vi "Get Count LED Settings From Recipe.vi"(11 "Test Recipe in":refnum<class "Test Recipe.lvclass">) -> (1 "Threshold Values":T1={"Red Range"={"Lower value"=0, "Upper value"=95}, "Green Range"={"Lower value"=0, "Upper value"=95}, "Blue Range"={"Lower value"=115, "Upper value"=255}}, 2 "Rectangle":T2 {"Rotation" format="%.2f"; "Left" scale=0.0..1024.0; "Right" scale=0.0..1024.0}, 3 "Search Settings":T3, 4 "Minimum Artifact Size":dbl, 5 "Exposure Speed":dbl)   [LabVIEW 2015]
uses:
  Classes/Test Recipe/Class/Test Recipe.lvclass
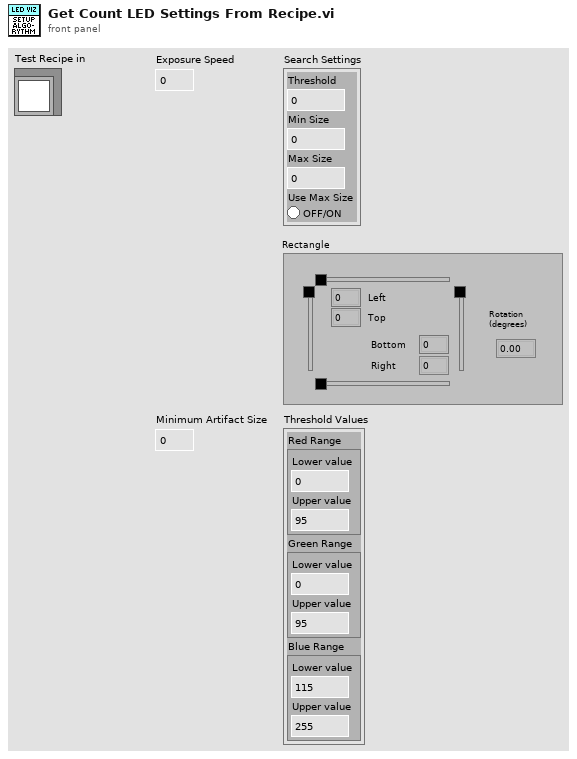
[diagram p1: front panel]
types:
  T1 = cluster{"Red Range":cluster{"Lower value":i32, "Upper value":i32}, "Green Range":cluster{"Lower value":i32, "Upper value":i32}, "Blue Range":cluster{"Lower value":i32, "Upper value":i32}}
  T2 = typedef "IMAQ Rectangle" = cluster{"Left":i32, "Top":i32, "Right":i32, "Bottom":i32, "Rotation":dbl}
  T3 = cluster{"Threshold":u32, "Min Size":u32, "Max Size":u32, "Use Max Size":bool}
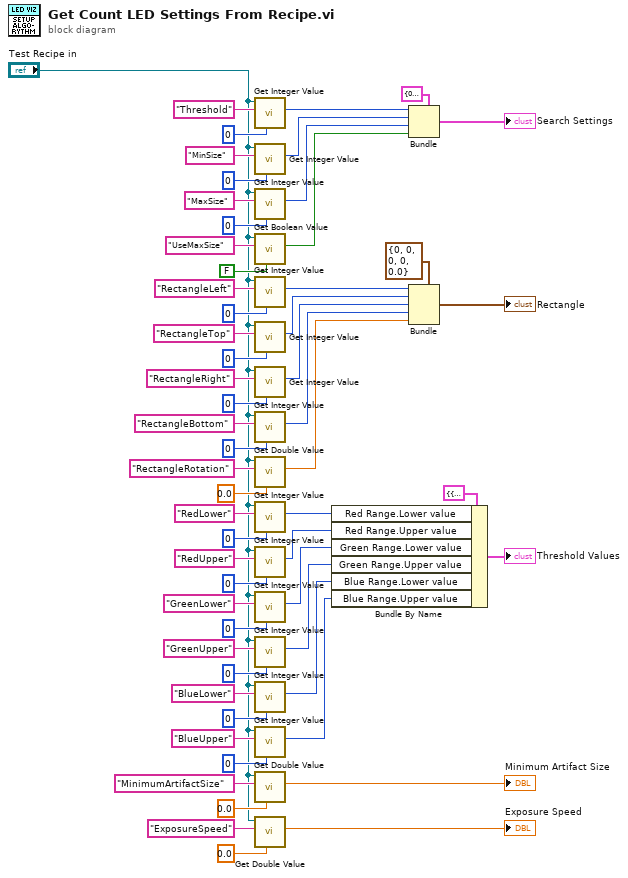
[diagram p0: block diagram]
diagram:
  n1 = call "Get Integer Value.vi"("Default Value"=u32 0, "Name"="Threshold", "Test Recipe in"="Test Recipe in") -> ("Value"=w48:i32)  [unwired: 5 in, 3 out]
  n2 = call "Get Integer Value.vi"("Default Value"=u32 0, "Name"="MinSize", "Test Recipe in"="Test Recipe in") -> ("Value"=w47:i32)  [unwired: 5 in, 3 out]
  n3 = call "Get Integer Value.vi"("Default Value"=u32 0, "Name"="MaxSize", "Test Recipe in"="Test Recipe in") -> ("Value"=w46:i32)  [unwired: 5 in, 3 out]
  n4 = call "Get Boolean Value.vi"("Default Value"=FALSE, "Name"="UseMaxSize", "Test Recipe in"="Test Recipe in") -> ("Value"=w45:bool)  [unwired: 5 in, 3 out]
  n5 = call "Get Integer Value.vi"("Default Value"=u32 0, "Name"="RectangleLeft", "Test Recipe in"="Test Recipe in") -> ("Value"=w32:i32)  [unwired: 5 in, 3 out]
  n6 = call "Get Integer Value.vi"("Default Value"=u32 0, "Name"="RectangleTop", "Test Recipe in"="Test Recipe in") -> ("Value"=w31:i32)  [unwired: 5 in, 3 out]
  n7 = call "Get Integer Value.vi"("Default Value"=u32 0, "Name"="RectangleRight", "Test Recipe in"="Test Recipe in") -> ("Value"=w30:i32)  [unwired: 5 in, 3 out]
  n8 = call "Get Integer Value.vi"("Default Value"=u32 0, "Name"="RectangleBottom", "Test Recipe in"="Test Recipe in") -> ("Value"=w29:i32)  [unwired: 5 in, 3 out]
  n9 = call "Get Double Value.vi"("Default Value"=0.0, "Name"="RectangleRotation", "Test Recipe in"="Test Recipe in") -> ("Value"=w26:dbl)  [unwired: 5 in, 3 out]
  n10 = call "Get Integer Value.vi"("Default Value"=u32 0, "Name"="RedLower", "Test Recipe in"="Test Recipe in") -> ("Value"=w11:i32)  [unwired: 5 in, 3 out]
  n11 = call "Get Integer Value.vi"("Default Value"=u32 0, "Name"="RedUpper", "Test Recipe in"="Test Recipe in") -> ("Value"=w10:i32)  [unwired: 5 in, 3 out]
  n12 = call "Get Integer Value.vi"("Default Value"=u32 0, "Name"="GreenLower", "Test Recipe in"="Test Recipe in") -> ("Value"=w9:i32)  [unwired: 5 in, 3 out]
  n13 = call "Get Integer Value.vi"("Default Value"=u32 0, "Name"="GreenUpper", "Test Recipe in"="Test Recipe in") -> ("Value"=w8:i32)  [unwired: 5 in, 3 out]
  n14 = call "Get Integer Value.vi"("Default Value"=u32 0, "Name"="BlueLower", "Test Recipe in"="Test Recipe in") -> ("Value"=w7:i32)  [unwired: 5 in, 3 out]
  n15 = call "Get Integer Value.vi"("Default Value"=u32 0, "Name"="BlueUpper", "Test Recipe in"="Test Recipe in") -> ("Value"=w6:i32)  [unwired: 5 in, 3 out]
  n16 = call "Get Double Value.vi"("Default Value"=0.0, "Name"="MinimumArtifactSize", "Test Recipe in"="Test Recipe in") -> ("Value"=→"Minimum Artifact Size":dbl)  [unwired: 5 in, 3 out]
  n17 = call "Get Double Value.vi"("Default Value"=0.0, "Name"="ExposureSpeed", "Test Recipe in"="Test Recipe in") -> ("Value"=→"Exposure Speed":dbl)  [unwired: 5 in, 3 out]
  n18 = Bundle By Name(cluster=T1 {"Red Range"={"Lower value"=0, "Upper value"=95}, "Green Range"={"Lower value"=0, "Upper value"=95}, "Blue Range"={"Lower value"=115, "Upper value"=255}} ("Threshold Values"), "Red Range.Lower value"=w11, "Red Range.Upper value"=w10, "Green Range.Lower value"=w9, "Green Range.Upper value"=w8, "Blue Range.Lower value"=w7, "Blue Range.Upper value"=w6) -> (→"Threshold Values":T1)
  n19 = Bundle(cluster=T3 {"Threshold"=0, "Min Size"=0, "Max Size"=0, "Use Max Size"=FALSE}, "Threshold"=w48, "Min Size"=w47, "Max Size"=w46, "Use Max Size"=w45) -> (→"Search Settings":T3)
  n20 = Bundle(cluster=T2 {"Left"=0, "Top"=0, "Right"=0, "Bottom"=0, "Rotation"=0.0} ("Rectangle"), "Left"=w32, "Top"=w31, "Right"=w30, "Bottom"=w29, "Rotation"=w26) -> (→"Rectangle":T2)
